vi "avalibale printers.vi"(8 "error in (no error)":errorcluster) -> (0 "error out":errorcluster, 1 "Printing:Available Printers":string[](array[string]), 3 "Printing:Default Printer":string)   [LabVIEW 2013]
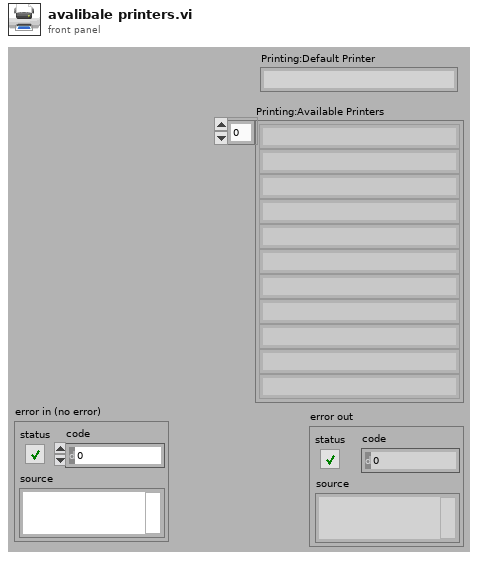
[diagram p1: front panel]
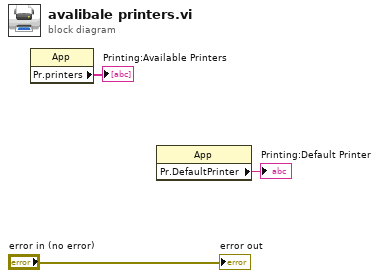
[diagram p0: block diagram]
diagram:
  n1 = property class="App"() -> ("Pr.printers"=→"Printing:Available Printers":string[])  [unwired: 2 in, 2 out]
  n2 = property class="App"() -> ("Pr.DefaultPrinter"=→"Printing:Default Printer":string)  [unwired: 2 in, 2 out]
  "error out" <- "error in (no error)"
